vi "Setup subWorker - TCP Listener.vi"(8 "error in":errorcluster, 11 "TCP Server in":refnum<class "DS TCP Server.lvclass">) -> (0 "error out":errorcluster, 3 "TCP Server out":refnum<class "DS TCP Server.lvclass">)   [LabVIEW 2017, in "DS TCP Server.lvlib" / "DS TCP Server.lvclass"]
doc: "<b>Note: Do not change the code in this VI!</b>\nThis VI performs a setup of all the statically-linked subWorkers that belong to the Worker that calls this VI. This VI is created automatically by the 'Create/Add Worker' tool and must be called <b>before</b> any statically linked subWorkers are called."
uses:
  DS TCP Server.lvclass
  DS TCP Server.lvclass/DS TCP Server.ctl
  DS TCP Listener/DS TCP Listener.lvclass
  C:/Program Files (x86)/National Instruments/LabVIEW 2017/vi.lib/addons/_Workers/Library/Classes/Worker/Worker.lvclass
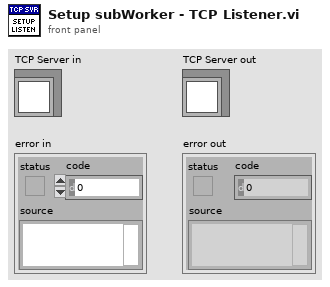
[diagram p1: front panel]
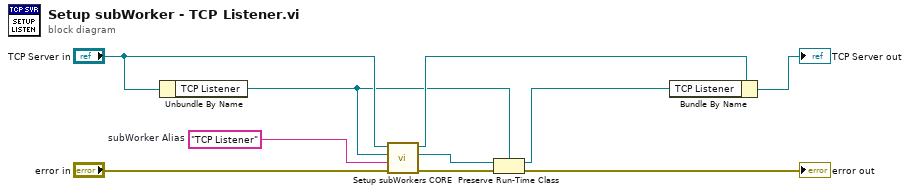
[diagram p0: block diagram]
diagram:
  w6 = "TCP Listener"  # subWorker Alias
  n1 = Unbundle By Name("TCP Server in") -> ("TCP Listener"=w3:refnum<class "DS TCP Listener.lvclass">)
  n2 = call-dynamic "Setup subWorkers CORE.vi"("error in"="error in", "subWorker Alias"=w6, "subWorker"=w3, "Worker"="TCP Server in") -> ("error out"=w5:errorcluster, "subWorker out"=w1:refnum<class "Worker.lvclass">, "Worker out"=w8:refnum<class "DS TCP Server.lvclass">)  [unwired: 5 in]
  n3 = Preserve Run-Time Class(object in=w1, error in=w5, 2:w3) -> (object out=w2:refnum<class "DS TCP Listener.lvclass">, error out=→"error out":errorcluster)
  n4 = Bundle By Name(cluster=w8, "TCP Listener"=w2) -> (→"TCP Server out":refnum<class "DS TCP Server.lvclass">)
